vi "find immediate threats.vi"(10 "Maze (0: Empty, -1: Enemy. 1: Teammate":i32[][](array[numeric])) -> (1 "My square?":bool, 2 "threats?":bool)   [LabVIEW 2014, in "JFD_Common.lvlib"]
uses:
  JFD_Common.lvlib
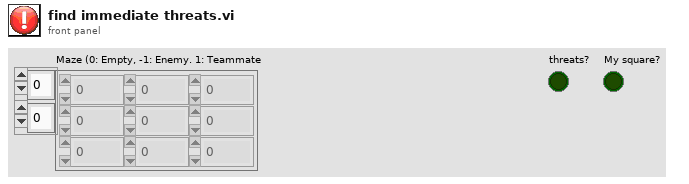
[diagram p1: front panel]
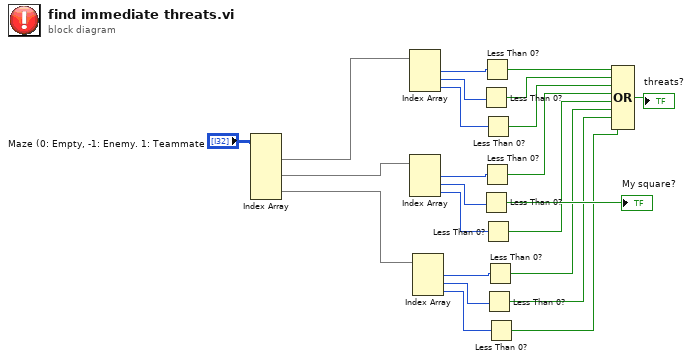
[diagram p0: block diagram]
diagram:
  n1 = Index Array(array="Maze (0: Empty, -1: Enemy. 1: Teammate") -> (element #1=w22:i32[], element #2=w12:i32[], element #3=w11:i32[])  [unwired: 6 in]
  n2 = Index Array(array=w22) -> (element #1=w21:i32, element #2=w20:i32, element #3=w19:i32)  [unwired: 3 in]
  n3 = Index Array(array=w12) -> (element #1=w16:i32, element #2=w17:i32, element #3=w18:i32)  [unwired: 3 in]
  n4 = Index Array(array=w11) -> (element #1=w15:i32, element #2=w14:i32, element #3=w13:i32)  [unwired: 3 in]
  n5 = Less Than 0?(x=w20) -> (x < 0?=w9:bool)
  n6 = Less Than 0?(x=w17) -> (x < 0?=→"My square?":bool)
  n7 = Less Than 0?(x=w21) -> (x < 0?=w10:bool)
  n8 = Less Than 0?(x=w16) -> (x < 0?=w7:bool)
  n9 = Less Than 0?(x=w19) -> (x < 0?=w8:bool)
  n10 = Less Than 0?(x=w18) -> (x < 0?=w5:bool)
  n11 = Less Than 0?(x=w14) -> (x < 0?=w3:bool)
  n12 = Less Than 0?(x=w15) -> (x < 0?=w4:bool)
  n13 = Less Than 0?(x=w13) -> (x < 0?=w2:bool)
  n14 = Compound Arithmetic op=OR(w10, w9, w8, w7, w5, w4, w3, w2) -> (→"threats?":bool)
